vi "Arc_to_Points.vi"(10 "Data Matrix":T1=[[50.0, 50.0, 0.0, 1.0, 0.0, 0.0, 0.0], [100.0, 50.0, 0.0, 2.0, 75.0, 75.0, 0.0], [100.0, 100.0, 0.0, 1.0, 0.0, 0.0, 0.0], [50.0, 100.0, 0.0, 1.0, 0.0, 0.0, 0.0]]) -> (2 "Points of Data Matrix":dbl[][](array[numeric]))   [LabVIEW 2014]
doc: "读取各个点的数据"
uses:
  <vilib>/Analysis/Matrix/Datatypes/RealMatrix.ctl
  <vilib>/Analysis/Matrix/Numeric/Conversions/Matrix To Array - RM.vi
  <vilib>/Analysis/Matrix/NI_Matrix.lvlib
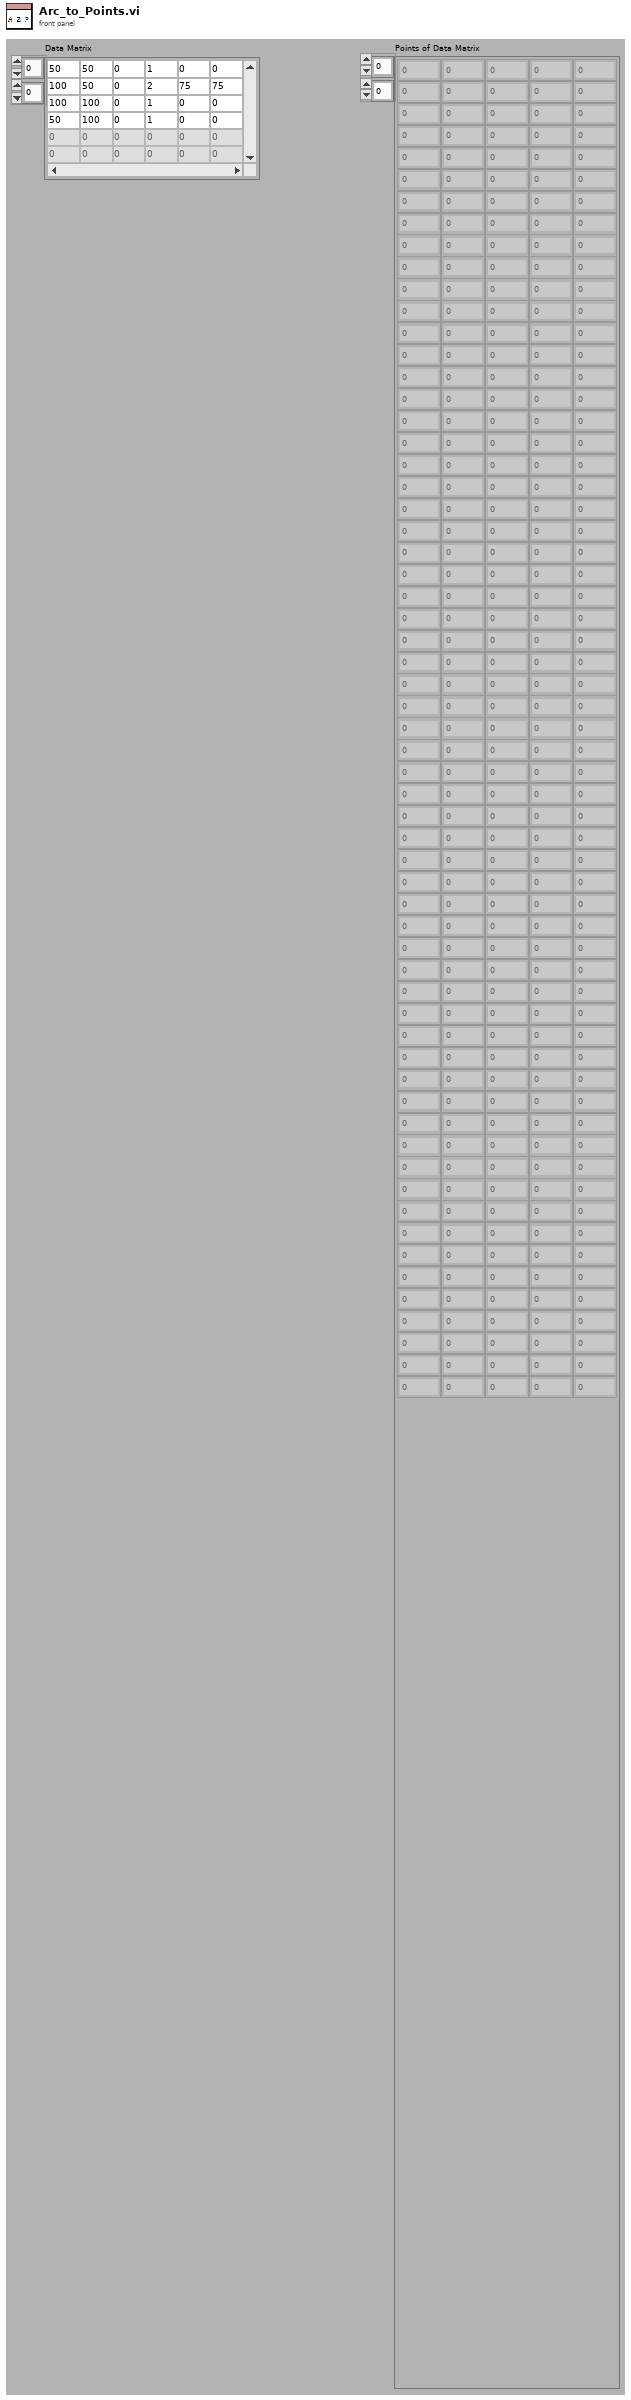
[diagram p1: front panel]
types:
  T1 = typedef "NI_Matrix.lvlib/RealMatrix.ctl" = dbl[][]
  T2 = cluster{"Real Matrix Element":dbl, "Real Matrix Element":dbl}
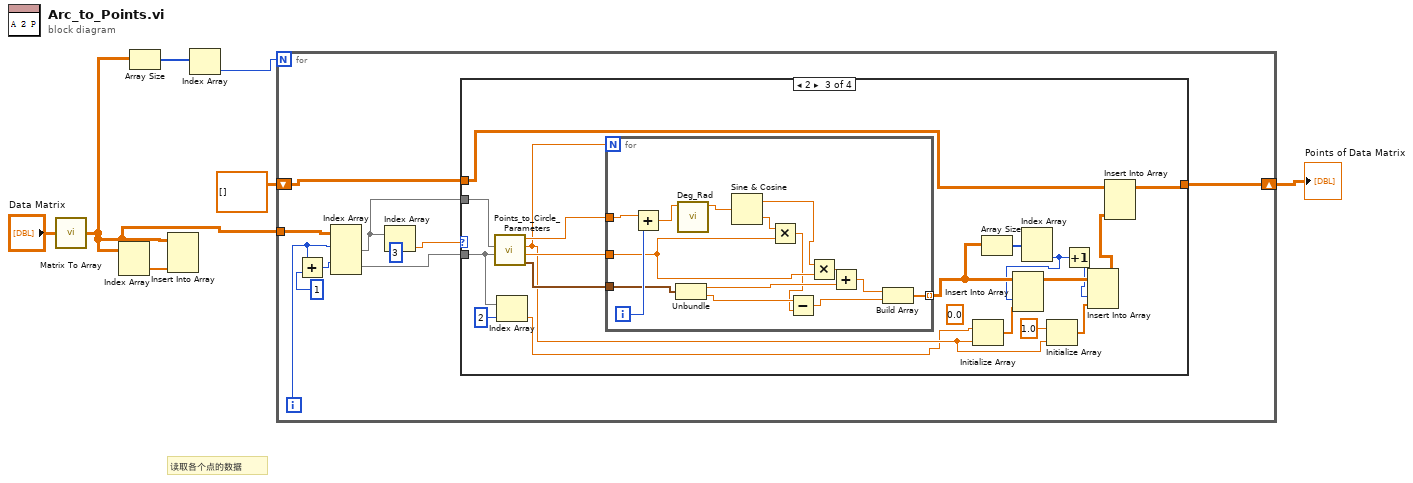
[diagram p0: block diagram]
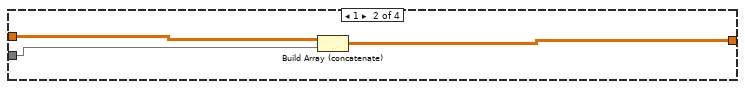
[diagram p3: hidden frame]
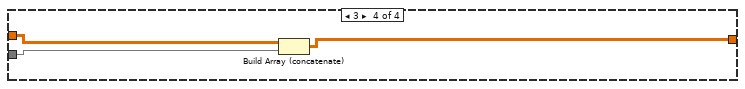
[diagram p4: hidden frame]
diagram:
  # "读取各个点的数据"
  n1 = call-poly <vilib>:"Matrix To Array.vi"("Real Matrix"="Data Matrix") -> ("Real 2D Array"=w1:dbl[][])
  n2 = Index Array(array=w1) -> (element=w2:dbl[])  [unwired: 2 in]
  n3 = Array Size(array=w1) -> (size(s)=w6:i32[])
  n4 = Insert Into Array(array=w1, new element=w2) -> ()  [unwired: 2 in, 1 out]
  n5 = Index Array(array=w6) -> (element=w5:i32)  [unwired: 1 in]
  n6 = for {
    N: w5 -> [_]
    tunnel: w1 -> [w15]
    shift-right: [w12] -> w3
    shift-left: dbl[][] [] -> [w11]
    i -> [w8]
    n7 = Add(x=w8, y=1) -> (x+y=w17:i32)
    n8 = Index Array(array=w15, index (row) #1=w8, index (row) #2=w17) -> (element #1=w13:dbl[], element #2=w10:dbl[])  [unwired: 2 in]
    n9 = Index Array(array=w13, index=3 ("索引")) -> (element=w14:dbl)
    n10 = case shown="2" w14 {
      tunnel: w13 -> [_ w19 w40 w57]
      tunnel: [w18 w21 w34 w56] -> w12
      tunnel: w11 -> [w18 w20 w35 w58]
      tunnel: w10 -> [_ _ w24 _]
      frame 0, Default {
      }
      frame 1 {
        n11 = Build Array (concatenate)(w20, w19) -> (w21:dbl[][])
      }
      frame 2 {
        (unwired) 0.0 ("元素")
        n12 = call "Points_to_Circle_Parameters.vi"("Arc End point"=w24, "Arc Start point"=w40) -> ("Center point"=w37:T2, "Radius"=w39:dbl, "Center Deg"=w30:dbl, "Start Deg"=w38:dbl)  [unwired: 6 in]
        n13 = Index Array(array=w24, index=2 ("索引")) -> (element=w22:dbl)
        n14 = for {
          N: w30 -> [_]
          tunnel: w39 -> [w46]
          tunnel: w38 -> [w55]
          tunnel: w37 -> [w51]
          tunnel: [w41] -> w28 mode=indexing
          i -> [w54]
          n15 = Add(x=w55, y=w54) -> (x+y=w53:dbl)
          n16 = Unbundle(w51) -> ("Real Matrix Element"=w48:dbl, "Real Matrix Element"=w45:dbl)
          n17 = call "Deg_Rad.vi"("Deg"=w53) -> ("Rad"=w52:dbl)  [unwired: 9 in, 1 out]
          n18 = Sine & Cosine(0:w52) -> (1:w50:dbl, 2:w47:dbl)
          n19 = Multiply(x=w47, y=w46) -> (x*y=w44:dbl)
          n20 = Subtract(x=w45, y=w44) -> (x-y=w42:dbl)
          n21 = Multiply(x=w50, y=w46) -> (x*y=w49:dbl)
          n22 = Add(x=w49, y=w48) -> (x+y=w43:dbl)
          n23 = Build Array(w43, w42) -> (w41:dbl[])
        }
        n24 = Initialize Array(w22, w30) -> (w36:dbl[])
        n25 = Array Size(array=w28) -> (size(s)=w27:i32[])
        n26 = Index Array(array=w27) -> (element #2=w26:i32)  [unwired: 2 in, 1 out]
        n27 = Insert Into Array(array=w28, index (col)=w26, new element=w36) -> (w33:dbl[][])  [unwired: 1 in]
        n28 = Initialize Array(1.0 ("元素"), w30) -> (w31:dbl[])
        n29 = Increment(x=w26) -> (x+1=w25:i32)
        n30 = Insert Into Array(array=w33, index (col)=w25, new element=w31) -> (w29:dbl[][])  [unwired: 1 in]
        n31 = Insert Into Array(array=w35, new element=w29) -> (w34:dbl[][])  [unwired: 2 in]
      }
      frame 3 {
        n32 = Build Array (concatenate)(w58, w57) -> (w56:dbl[][])
      }
    }
  }
  "Points of Data Matrix" <- w3
